vi "Sort by 2nd element.vi"(10 "correspondence table in":T1 {"volts" format="%.4f"; "physical units" format="%.4f"}) -> (3 "correspondence table out":T1 {"volts" format="%.4f"; "physical units" format="%.4f"})   [LabVIEW 2019]
uses:
  correspondence table.ctl
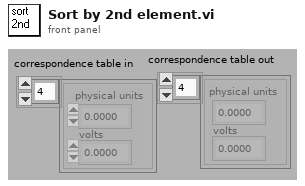
[diagram p1: front panel]
types:
  T1 = typedef "correspondence table.ctl" = cluster{"physical units":dbl, "volts":dbl}[]
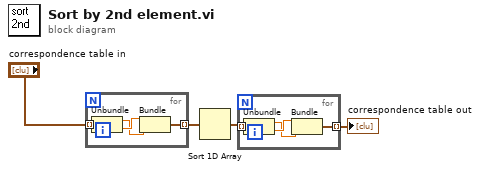
[diagram p0: block diagram]
diagram:
  n1 = for {
    tunnel: "correspondence table in" -> [w8] mode=indexing
    tunnel: [w5] -> w3 mode=indexing
    n2 = Unbundle(w8) -> ("physical units"=w6:dbl, "volts"=w7:dbl)
    n3 = Bundle("volts"=w7, "physical units"=w6) -> (w5:cluster{"volts":dbl, "physical units":dbl})  [unwired: 1 in]
  }
  n4 = Sort 1D Array(array=w3) -> (sorted array=w2:cluster{"volts":dbl, "physical units":dbl}[])
  n5 = for {
    tunnel: w2 -> [w12] mode=indexing
    tunnel: [w9] -> w1 mode=indexing
    n6 = Unbundle(w12) -> ("volts"=w10:dbl, "physical units"=w11:dbl)
    n7 = Bundle("physical units"=w11, "volts"=w10) -> (w9:cluster{"physical units":dbl, "volts":dbl})  [unwired: 1 in]
  }
  "correspondence table out" <- w1
